vi "BeamGage Chart.vi"() -> ()   [LabVIEW 2009]
uses:
  C:/Program Files/Spiricon/BeamGage Professional/Spiricon.BeamGage.Automation.dll
panel:
  out "2D Intensity Graph":dbl[][](graph)
  out "1D Profile - Peak Location Y - Waveform Graph":dbl[](graph)
  out "Height":dbl
  out "Width":dbl
  out "Peak Loc Y":dbl
  out "Peak Loc X":dbl
  in  "START_STOP":bool
  in  "ULTRACAL":bool
  out "Total and Peak Power - Waveform Chart":cluster{"Total":dbl, "Peak":dbl}(graph)
  in  "STOP SERVER":bool
  # "Block laser beam and \nclick Ultracal to calibrate"
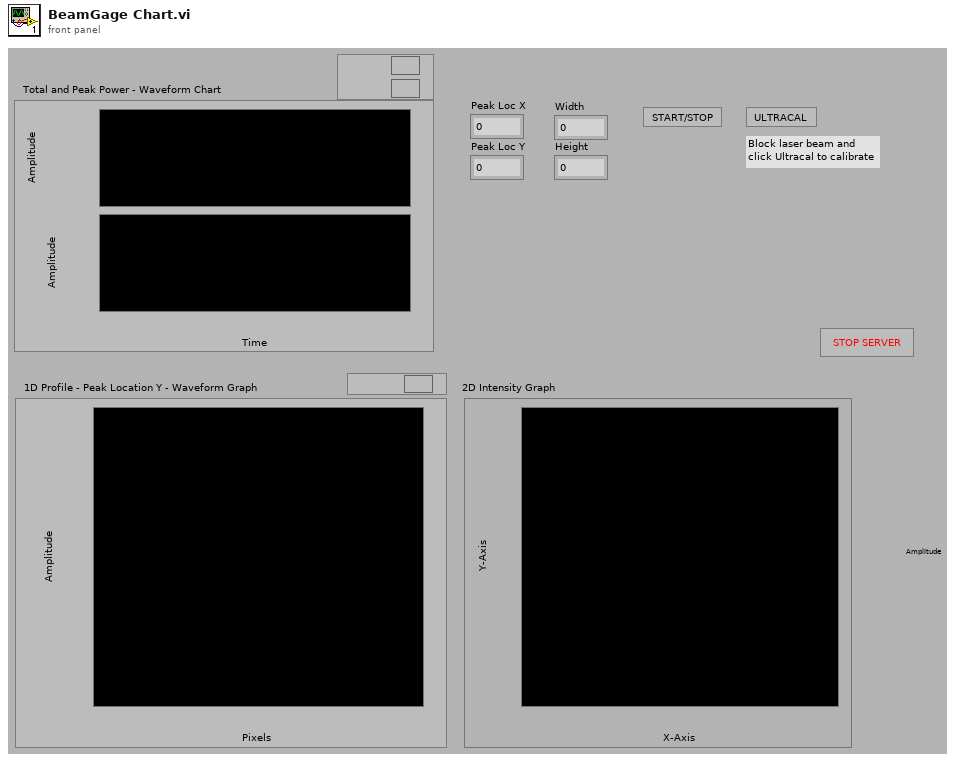
[diagram p1: front panel]
types:
  T1 = cluster{"Total":dbl, "Peak":dbl, "Peak X":dbl, "Peak Y":dbl, "Width":dbl, "Height":dbl, "DoubleData":dbl[]}
  T2 = cluster{"notifier out":refnum<notifier>, "new reference":refnum<k24>}
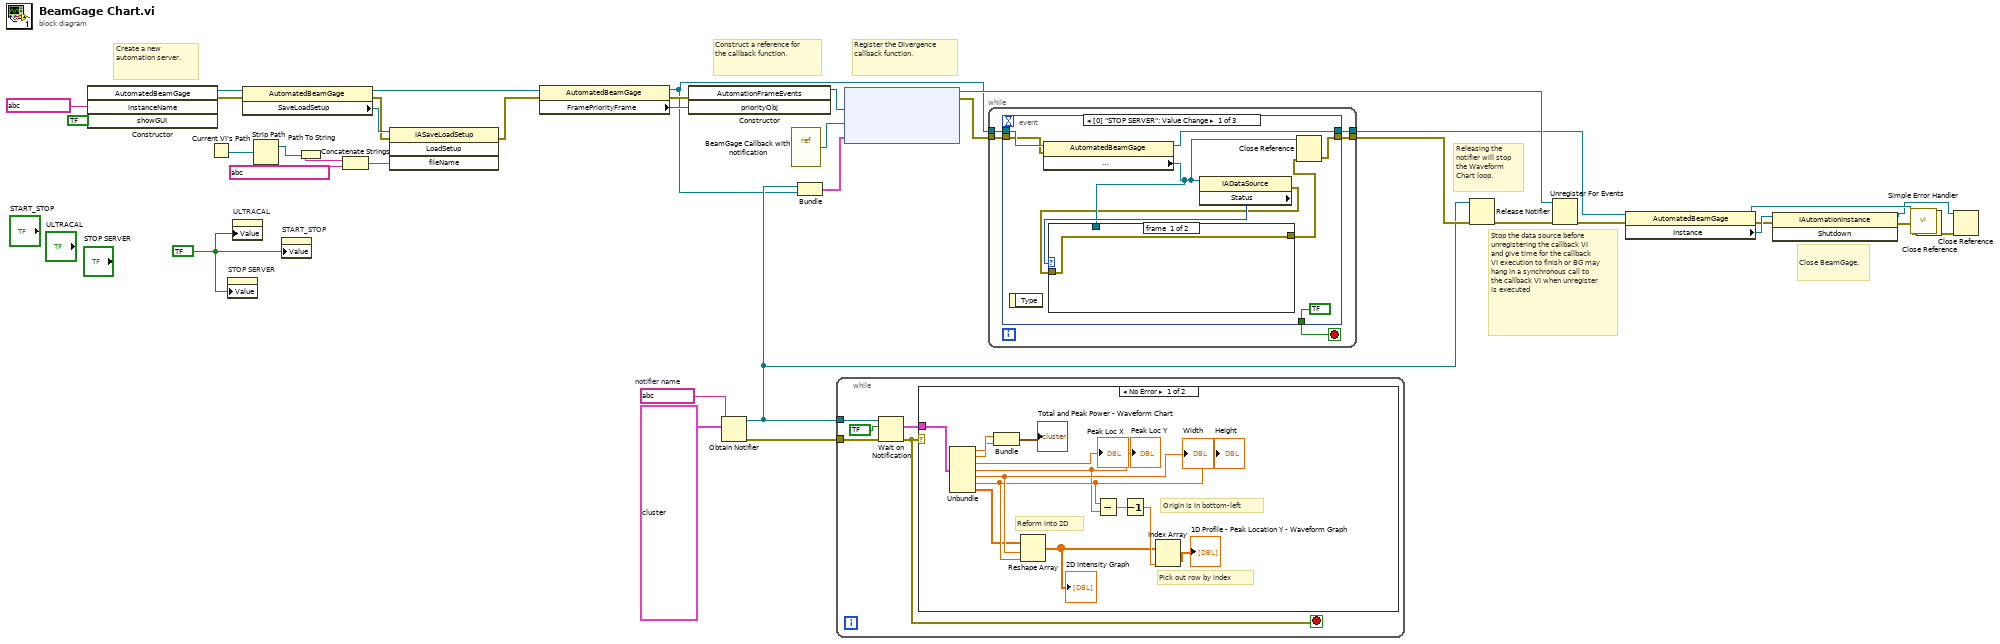
[diagram p0: block diagram]
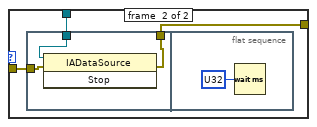
[diagram p2: hidden frame]
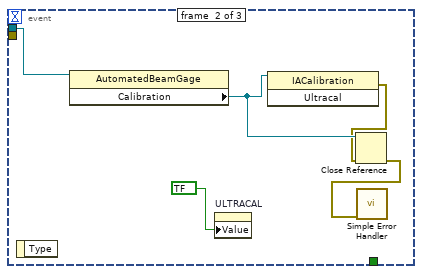
[diagram p3: hidden frame]
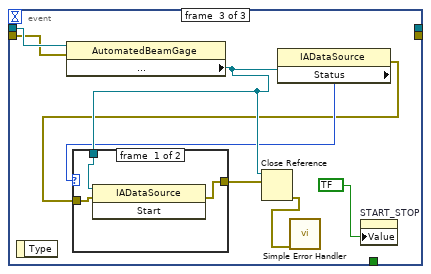
[diagram p4: hidden frame]
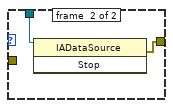
[diagram p5: hidden frame]
diagram:
  w34 = bool ? ("stop")
  w37 = string ?  # notifier name
  # "Stop the data source before unregistering the callback VI  and give time for the callback VI execution to finish or BG may hang in a synchronous call to the callback VI when unregister is executed"
  # "Releasing the notifier will stop the Waveform Chart loop."
  # "Close BeamGage."
  # "Create a new automation server."
  # "Register the Divergence callback function."
  # "Construct a reference for the callback function."
  n1 = constructor class="AutomatedBeamGage"("instanceName"=string ?, "showGUI"=bool ?) -> (reference out=w10:refnum<k24>, error out=w11:errorcluster)  [unwired: 3 in, 3 out]
  n2 = Current VI's Path() -> (path=w3:path)
  n3 = property on="STOP SERVER" class="Bool (strict)"("Value"=w34) -> ()  [unwired: 2 in, 2 out]
  n4 = property on="ULTRACAL" class="Bool (strict)"("Value"=w34) -> ()  [unwired: 2 in, 2 out]
  n5 = property class="AutomatedBeamGage"(reference=w10, error in=w11) -> (reference out=w6:refnum<k24>, error out=w8:errorcluster, "SaveLoadSetup"=w9:refnum<k24>)
  n6 = Strip Path(path=w3) -> (stripped path=w2:path)  [unwired: 1 out]
  n7 = property on="START_STOP" class="Bool (strict)"("Value"=w34) -> ()  [unwired: 2 in, 2 out]
  n8 = Path To String(path=w2) -> (string=w5:string)
  n9 = Concatenate Strings(w5, string ? ("string")) -> (w1:string)
  n10 = invoke class="IASaveLoadSetup" method="LoadSetup"(reference=w9, error in=w8, "fileName"=w1) -> (error out=w7:errorcluster)  [unwired: 1 in, 3 out]
  n11 = property class="AutomatedBeamGage"(reference=w6, error in=w7) -> (reference out=w15:refnum<k24>, error out=w17:errorcluster, "FramePriorityFrame"=w18:refnum<k24>)
  n12 = constructor class="AutomationFrameEvents"(error in=w17, "priorityObj"=w18) -> (reference out=w16:refnum<k24>)  [unwired: 2 in, 3 out]
  n13 = Obtain Notifier(name (unnamed)=w37, notification data type=T1 ?) -> (notifier out=w29:refnum<notifier>, error out=w35:errorcluster)  [unwired: 2 in, 1 out]
  n14 = vi-ref "BeamGage Callback with notification.vi"() -> (w24:refnum<vi>)
  n15 = Bundle("notifier out"=w29, "new reference"=w15) -> (w25:T2)  [unwired: 1 in]
  n16 = while {
    tunnel: w29 -> [w42]
    tunnel: w35 -> [w40]
    stop <- w38 stop-if-true
    n17 = Wait on Notification(notifier=w42, ignore previous (F)=bool ?, error in (no error)=w40) -> (notification=w41:T1, error out=w38:errorcluster)  [unwired: 1 in, 2 out]
    n18 = case shown="No Error" w38 {
      tunnel: w41 -> [w55 _]
      frame #0 {
        # "Pick out row by index"
        # "Reform into 2D"
        # "Origin is in bottom-left"
        n19 = Unbundle(w55) -> ("Total"=w54:dbl, "Peak"=w53:dbl, "Peak X"=→"Peak Loc X":dbl, "Peak Y"=w47:dbl, "Width"=w50:dbl, "Height"=w48:dbl, "DoubleData"=w44:dbl[])
        "Peak Loc Y" <- w47
        "Width" <- w50
        "Height" <- w48
        n20 = Bundle("Total"=w54, "Peak"=w53) -> (→"Total and Peak Power - Waveform Chart":cluster{"Total":dbl, "Peak":dbl})  [unwired: 1 in]
        n21 = Reshape Array(w44, w50, w48) -> (w43:dbl[][])
        "2D Intensity Graph" <- w43
        n22 = Subtract(x=w48, y=w47) -> (x-y=w49:dbl)
        n23 = Decrement(x=w49) -> (x-1=w46:dbl)
        n24 = Index Array(array=w43, index (col)=w46) -> (element=→"1D Profile - Peak Location Y - Waveform Graph":dbl[])  [unwired: 1 in]
      }
      frame #1 {
        # "Don't update chart when an error occurs."
      }
    }
  }
  n25 = node(w16, w24, w25) -> (w33:refnum<k27>, w31:errorcluster)  [unwired: 2 in]
  n26 = while {
    tunnel: [w60] -> w23
    tunnel: w15 -> [w59]
    tunnel: w31 -> [w57]
    tunnel: [w56] -> w30
    stop <- w58 stop-if-true
    n27 = event shown="[0] \"STOP SERVER\": Value Change" {
      selector: _ -> [_ _ _]
      dyn-events: _ -> [_ _ _]
      timeout: _ -> [_ _ _]
      tunnel: w59 -> [w67 w80 w87]
      tunnel: [w66 _ _] -> w60
      tunnel: [bool ? ("stop") _ _] -> w58
      tunnel: w57 -> [w65 _ w86]
      tunnel: [w68 _ _] -> w56
      event #0 {
        n28 = event-data() -> ()  [unwired: 1 in, 1 out]
        n29 = property class="AutomatedBeamGage"(reference=w67, error in=w65) -> (reference out=w66:refnum<k24>, "DataSource"=w63:refnum<k24>)  [unwired: 1 out]
        n30 = property class="IADataSource"(reference=w63) -> (error out=w61:errorcluster, "Status"=w64:i32)  [unwired: 1 in, 1 out]
        n31 = case shown="1" w64 {
          tunnel: w63 -> [_ w73]
          tunnel: [w70 w72] -> w62
          tunnel: w61 -> [w70 w71]
          frame #0 {
          }
          frame #1 {
            n32 = flat-sequence {
              tunnel: w73 -> [w76]
              tunnel: [w75] -> w72
              tunnel: w71 -> [w74]
              frame #0 {
                n33 = invoke class="IADataSource" method="Stop"(reference=w76, error in=w74) -> (error out=w75:errorcluster)  [unwired: 1 in, 2 out]
              }
              frame #1 {
                n34 = Wait (ms)(milliseconds to wait=u32 ?) -> ()  [unwired: 1 out]
              }
            }
          }
        }
        n35 = Close Reference(reference=w63, error in (no error)=w62) -> (error out=w68:errorcluster)
      }
      event #1 {
        n36 = event-data() -> ()  [unwired: 1 in, 1 out]
        n37 = property class="AutomatedBeamGage"(reference=w80) -> ("Calibration"=w79:refnum<k24>)  [unwired: 1 in, 2 out]
        n38 = property on="ULTRACAL" class="Bool (strict)"("Value"=bool ? ("stop")) -> ()  [unwired: 2 in, 2 out]
        n39 = invoke class="IACalibration" method="Ultracal"(reference=w79) -> (error out=w78:errorcluster)  [unwired: 2 in, 2 out]
        n40 = Close Reference(reference=w79, error in (no error)=w78) -> (error out=w81:errorcluster)
        n41 = call <vilib>:"Simple Error Handler.vi"("error in (no error)"=w81) -> ()  [unwired: 4 in, 5 out]
      }
      event #2 {
        n42 = event-data() -> ()  [unwired: 1 in, 1 out]
        n43 = property class="AutomatedBeamGage"(reference=w87, error in=w86) -> ("DataSource"=w85:refnum<k24>)  [unwired: 2 out]
        n44 = property class="IADataSource"(reference=w85) -> (error out=w83:errorcluster, "Status"=w84:i32)  [unwired: 1 in, 1 out]
        n45 = case shown="1" w84 {
          tunnel: [w91 w95] -> w89
          tunnel: w85 -> [w93 w94]
          tunnel: w83 -> [w92 _]
          frame #0 {
            n46 = invoke class="IADataSource" method="Start"(reference=w93, error in=w92) -> (error out=w91:errorcluster)  [unwired: 1 in, 2 out]
          }
          frame #1 {
            n47 = invoke class="IADataSource" method="Stop"(reference=w94) -> (error out=w95:errorcluster)  [unwired: 2 in, 2 out]
          }
        }
        n48 = Close Reference(reference=w85, error in (no error)=w89) -> (error out=w88:errorcluster)
        n49 = call <vilib>:"Simple Error Handler.vi"("error in (no error)"=w88) -> ()  [unwired: 4 in, 5 out]
        n50 = property on="START_STOP" class="Bool (strict)"("Value"=bool ? ("stop")) -> ()  [unwired: 2 in, 2 out]
      }
    }
  }
  n51 = Release Notifier(notifier=w29, error in (no error)=w30) -> (error out=w32:errorcluster)  [unwired: 1 in, 2 out]
  n52 = Unregister For Events(event registration refnum=w33, error in=w32) -> (error out=w20:errorcluster)
  n53 = property class="AutomatedBeamGage"(reference=w23, error in=w20) -> (reference out=w21:refnum<k24>, error out=w19:errorcluster, "Instance"=w22:refnum<k24>)
  n54 = invoke class="IAutomationInstance" method="Shutdown"(reference=w22, error in=w19) -> (reference out=w12:refnum<k24>, error out=w26:errorcluster)  [unwired: 1 in, 1 out]
  n55 = Close Reference(reference=w21, error in (no error)=w26) -> (error out=w14:errorcluster)
  n56 = Close Reference(reference=w12, error in (no error)=w14) -> (error out=w13:errorcluster)
  n57 = call <vilib>:"Simple Error Handler.vi"("error in (no error)"=w13) -> ()  [unwired: 4 in, 5 out]
